vi "SMTP Email Send File.vi"(0 "recipients":string[](array[string]), 1 "mail server":string, 2 "return address":string, 5 "subject ([No Subject])":string="[No Subject]", 7 "message":string, 9 "file path":path, 11 "error in (no error)":errorcluster, 12 "binary? (F)":bool, 13 "MIME content-type (application/octet-stream)":string="application/octet-stream") -> (4 "invalid recipients":string[](array[string]), 15 "error out":errorcluster)   [LabVIEW 2009, in "NewNI_SMTPEmail.lvlib"]
doc: "Sends an email with an attached file to a list of recipients."
uses:
  NewNI_SMTPEmail.lvlib
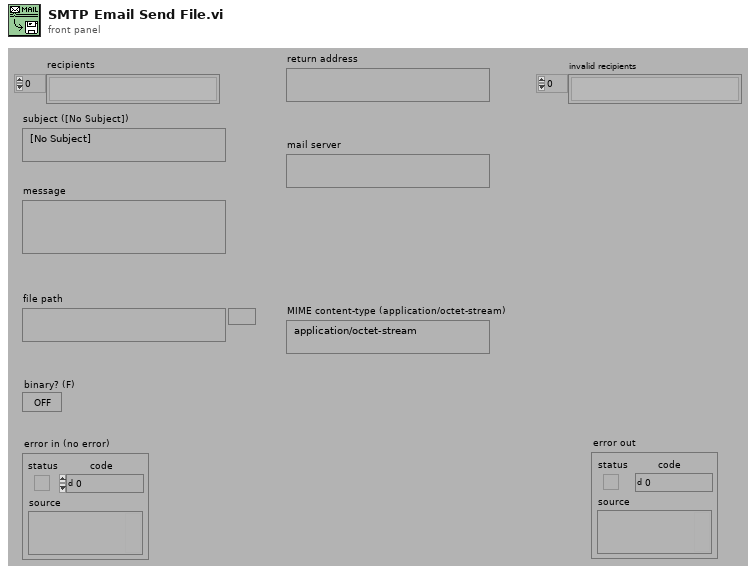
[diagram p1: front panel]
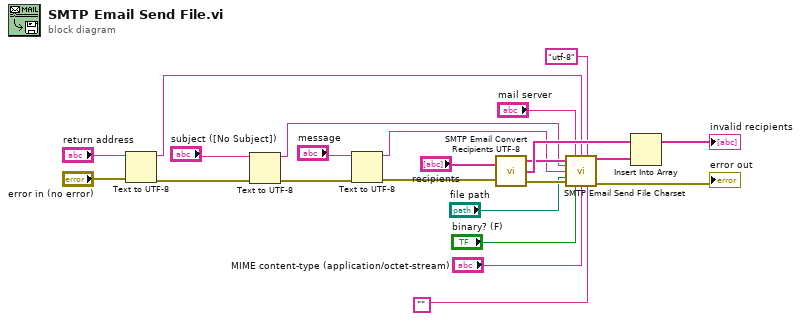
[diagram p0: block diagram]
diagram:
  n1 = Text to UTF-8(8:"error in (no error)", 11:"return address") -> (0:w18:errorcluster, 3:w8:string)
  n2 = Text to UTF-8(8:w18, 11:"subject ([No Subject])") -> (0:w20:errorcluster, 3:w6:string)
  n3 = Text to UTF-8(8:w20, 11:"message") -> (0:w22:errorcluster, 3:w5:string)
  n4 = call "SMTP Email Convert Recipients UTF-8.vi"("recipients"="recipients", "error in"=w22) -> ("convertible recipients"=w10:string[], "unconvertible recipients"=w12:string[], "error out"=w15:errorcluster)
  n5 = call "SMTP Email Send File Charset.vi"("recipients"=w10, "mail server"="mail server", "return address"=w8, "character set (us-ascii)"="utf-8", "subject ([No Subject])"=w6, "message"=w5, "file path"="file path", "error in (no error)"=w15, "binary? (F)"="binary? (F)", "MIME content-type (application/octet-stream)"="MIME content-type (application/octet-stream)", "translit"="") -> ("invalid recipients"=w16:string[], "error out"=→"error out":errorcluster)  [unwired: 3 out]
  n6 = Insert Into Array(array=w12, new element=w16) -> (→"invalid recipients":string[])  [unwired: 1 in]
